vi "Actor Core.vi"(8 "error in":errorcluster, 11 "ResultsViewer in":refnum<class "ResultsViewer.lvclass">) -> (0 "error out":errorcluster, 3 "Actor out":refnum<class "Actor.lvclass">)   [LabVIEW 2019, in "ResultsViewer.lvlib" / "ResultsViewer.lvclass"]
doc: "(<B>Filename</B>: Actor Framework.lvlib:Actor.lvclass:Actor Core.vi)\n\nReceives messages to the actor, reacts to them, and initiates any error handling that may shut the actor down.\n\nDescendant classes may override this VI to append parallel tasks for the actor to complete while it handles messages. Overrides use the Call Parent Class Method node."
uses:
  ResultsViewer.lvclass
  C:/Program Files (x86)/National Instruments/LabVIEW 2019/vi.lib/ActorFramework/Actor/Actor.lvclass
  <vilib>/ActorFramework/Actor/Actor.lvclass
  ResultsViewer.lvclass/ResultsViewer.ctl
  <vilib>/ActorFramework/Actor/Actor.lvclass/Actor.ctl
  <vilib>/ActorFramework/Message Enqueuer/Message Enqueuer.lvclass/Message Enqueuer.ctl
  <vilib>/ActorFramework/Message Enqueuer/Init from Existing Queue.vi
  <vilib>/ActorFramework/Message Enqueuer/Enqueue.vi
  <vilib>/ActorFramework/Stop Msg/Stop Msg.lvclass
  C:/Program Files (x86)/National Instruments/LabVIEW 2019/vi.lib/ActorFramework/Message/Message.lvclass
  <vilib>/Utility/LVClass/Get LV Class Name.vi
  <resource>/AFDebug/Generate Trace for Message.vi
  <vilib>/ActorFramework/Message Priority Queue/Priority Enqueue.vi
  <vilib>/ActorFramework/Message Enqueuer/Message Enqueuer.lvclass
panel:
  out "Loaded TDMS Filename":string
  out "O2 Saturation":dbl[](graph)
  out "Heart beat":dbl[](graph)
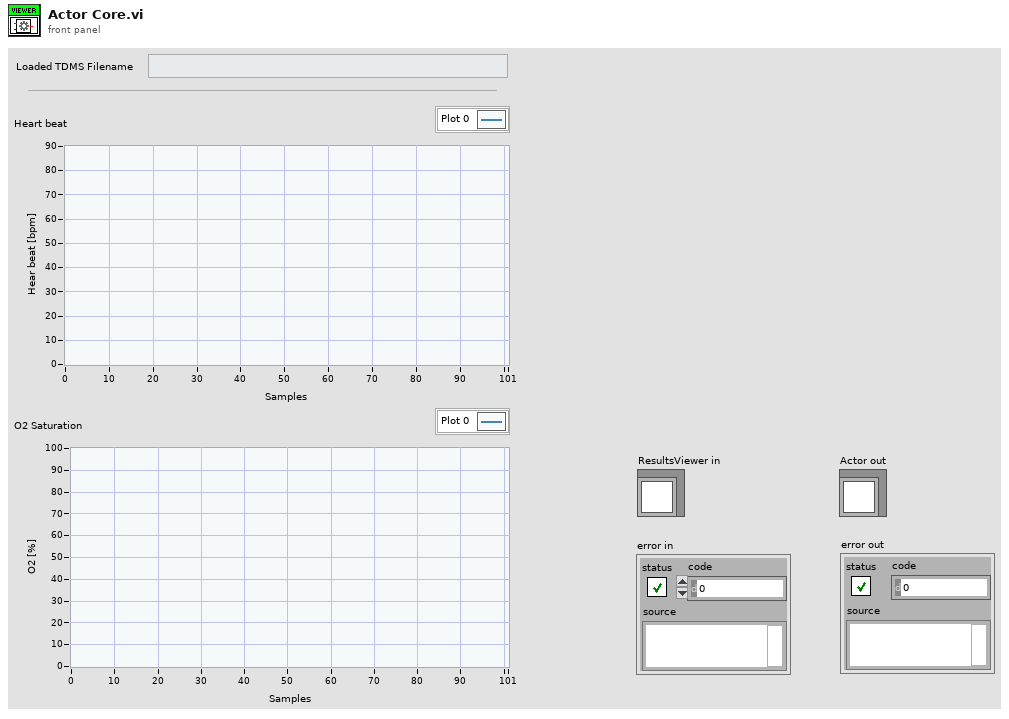
[diagram p1: front panel]
types:
  T1 = enum32{"Invalid", "Standard", "Closed", "Hidden", "Minimized", "Maximized"}
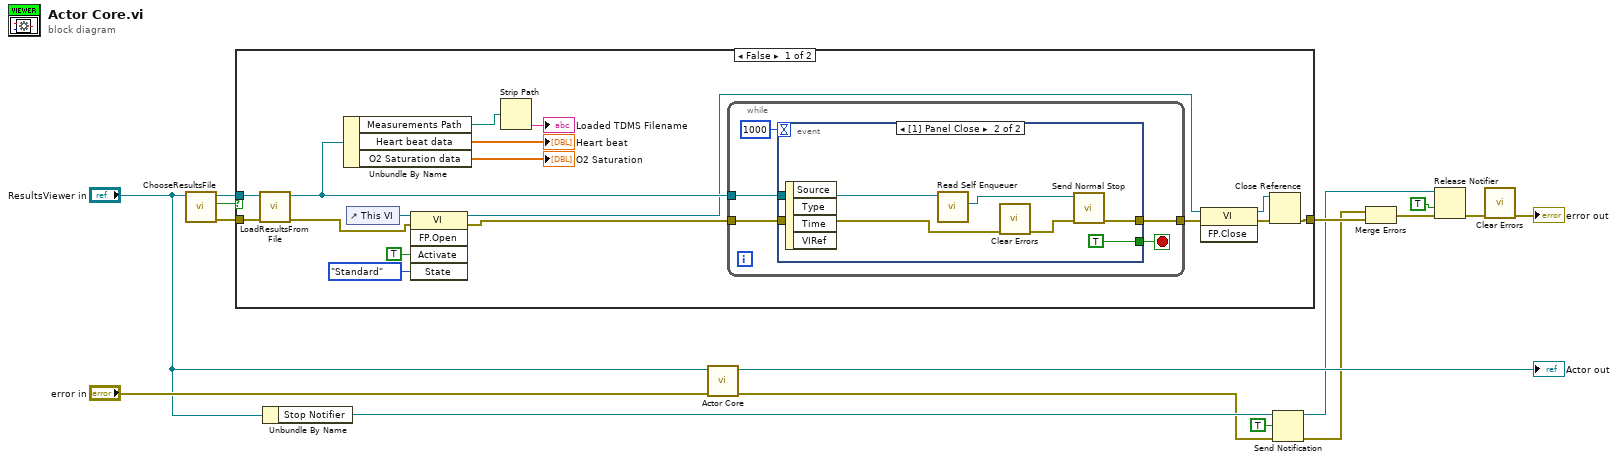
[diagram p0: block diagram]
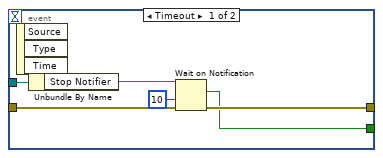
[diagram p2: hidden frame]
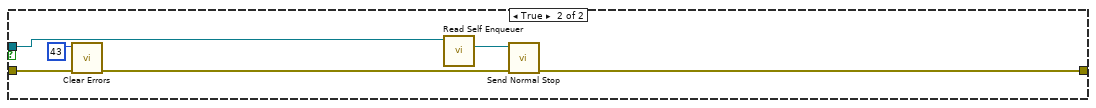
[diagram p3: hidden frame]
diagram:
  n1 = call "ChooseResultsFile.vi"("ResultsViewer in"="ResultsViewer in") -> ("error out"=w14:errorcluster, "Cancelled?"=w13:bool, "ResultsViewer out"=w15:refnum<class "ResultsViewer.lvclass">)  [unwired: 8 in]
  n2 = case shown="False" w13 {
    tunnel: w15 -> [w33 w55]
    tunnel: w14 -> [w32 w53]
    tunnel: [w18 w54] -> w12
    frame False {
      n3 = call "LoadResultsFromFile.vi"("error in (no error)"=w32, "ResultsViewer in"=w33) -> ("error out"=w23:errorcluster, "ResultsViewer out"=w31:refnum<class "ResultsViewer.lvclass">)  [unwired: 8 in]
      n4 = Unbundle By Name(w31) -> ("Measurements Path"=w28:path, "Heart beat data"=→"Heart beat":dbl[], "O2 Saturation data"=→"O2 Saturation":dbl[])
      n5 = control-ref of="This VI"() -> (w26:refnum<vi>)
      n6 = invoke class="VI" method="FP.Open"(reference=w26, error in=w23, "Activate"=TRUE ("Activate?"), "State"=T1."Standard") -> (reference out=w19:refnum<vi>, error out=w22:errorcluster)  [unwired: 1 in, 3 out]
      n7 = Strip Path(path=w28) -> (name=→"Loaded TDMS Filename":string)  [unwired: 1 out]
      n8 = while {
        tunnel: w22 -> [w37]
        tunnel: w31 -> [w38]
        tunnel: [w36] -> w21
        stop <- w35 stop-if-true
        n9 = event shown="[1] Panel Close" {
          selector: _ -> [_ _]
          dyn-events: _ -> [_ _]
          timeout: 1000 -> [_ _]
          tunnel: w38 -> [w43 w47]
          tunnel: w37 -> [w44 w48]
          tunnel: [w42 w46] -> w36
          tunnel: [w40 TRUE] -> w35
          event Timeout {
            n10 = event-data() -> ()  [unwired: 1 in, 3 out]
            n11 = Unbundle By Name(w43) -> ("Stop Notifier"=w41:refnum<notifier>)
            n12 = Wait on Notification(notifier=w41, timeout in ms (-1)=10, error in (no error)=w44) -> (notification=w40:bool, error out=w42:errorcluster)  [unwired: 1 in, 2 out]
          }
          event Panel Close {
            n13 = event-data() -> ()  [unwired: 1 in, 4 out]
            n14 = call <vilib>:"Read Self Enqueuer.vi"("Actor"=w47) -> ("Self Enqueuer"=w49:refnum<class "Message Enqueuer.lvclass">)  [unwired: 10 in]
            n15 = call <vilib>:"Clear Errors.vi"("error in (no error)"=w48) -> ("error out"=w45:errorcluster)  [unwired: 5 in, 1 out]
            n16 = call <vilib>:"Send Normal Stop.vi"("error in (no error)"=w45, "Message Enqueuer"=w49) -> ("error out"=w46:errorcluster)  [unwired: 9 in]
          }
        }
      }
      n17 = invoke class="VI" method="FP.Close"(reference=w19, error in=w21) -> (reference out=w17:refnum<vi>, error out=w20:errorcluster)  [unwired: 1 in, 1 out]
      n18 = Close Reference(reference=w17, error in (no error)=w20) -> (error out=w18:errorcluster)
    }
    frame True {
      n19 = call <vilib>:"Clear Errors.vi"("error in (no error)"=w53, "specific error code to clear (0: all)"=43) -> ("error out"=w52:errorcluster)  [unwired: 4 in, 1 out]
      n20 = call <vilib>:"Read Self Enqueuer.vi"("Actor"=w55) -> ("Self Enqueuer"=w56:refnum<class "Message Enqueuer.lvclass">)  [unwired: 10 in]
      n21 = call <vilib>:"Send Normal Stop.vi"("error in (no error)"=w52, "Message Enqueuer"=w56) -> ("error out"=w54:errorcluster)  [unwired: 9 in]
    }
  }
  n22 = Unbundle By Name("ResultsViewer in") -> ("Stop Notifier"=w7:refnum<notifier>)
  n23 = call-parent "Actor Core.vi"("error in"="error in", "Actor in"="ResultsViewer in") -> ("error out"=w5:errorcluster, "Actor out"=→"Actor out":refnum<class "Actor.lvclass">)  [unwired: 8 in]
  n24 = Send Notification(notification=TRUE, notifier=w7, error in (no error)=w5) -> (notifier out=w6:refnum<notifier>, error out=w4:errorcluster)
  n25 = Merge Errors(w4, w12) -> (w11:errorcluster)
  n26 = Release Notifier(notifier=w6, force destroy? (F)=TRUE, error in (no error)=w11) -> (error out=w8:errorcluster)  [unwired: 2 out]
  n27 = call <vilib>:"Clear Errors.vi"("error in (no error)"=w8) -> ("error out"=→"error out":errorcluster)  [unwired: 5 in, 1 out]
